vi "DecodeMonitorHeader(FHW0).vi"(11 "fhw0":u32 format="%.0x") -> (3 "FHW0":T1 {"MacID" format="%03b"})   [LabVIEW 2020, in "AIM664LV.lvlib"]
uses:
  AIM664LV.lvlib
  _controls/monitor_fhw0_type.ctl
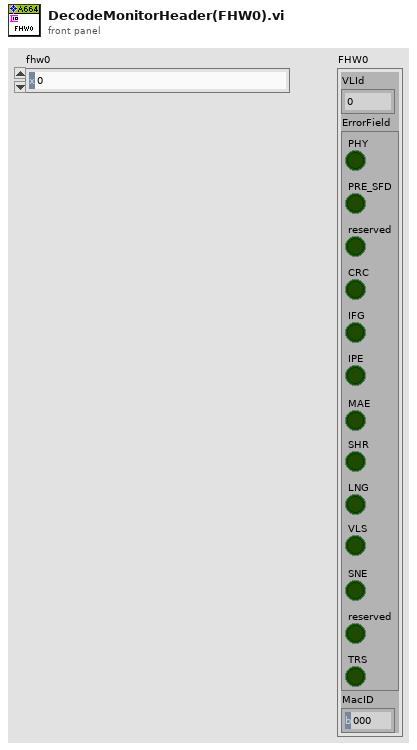
[diagram p1: front panel]
types:
  T1 = typedef "AIM664LV.lvlib/monitor_fhw0_type.ctl" = cluster{"VLId":u16, "ErrorField":cluster{"PHY":bool, "PRE_SFD":bool, "reserved":bool, "CRC":bool, "IFG":bool, "IPE":bool, "MAE":bool, "SHR":bool, "LNG":bool, "VLS":bool, "SNE":bool, "reserved":bool, "TRS":bool}, "MacID":u8}
  T2 = cluster{"Boolean array[0]":bool, "Boolean array[1]":bool, "Boolean array[2]":bool, "Boolean array[3]":bool, "Boolean array[4]":bool, "Boolean array[5]":bool, "Boolean array[6]":bool, "Boolean array[7]":bool, "Boolean array[8]":bool, "Boolean array[9]":bool, "Boolean array[10]":bool, "Boolean array[11]":bool, "Boolean array[12]":bool}
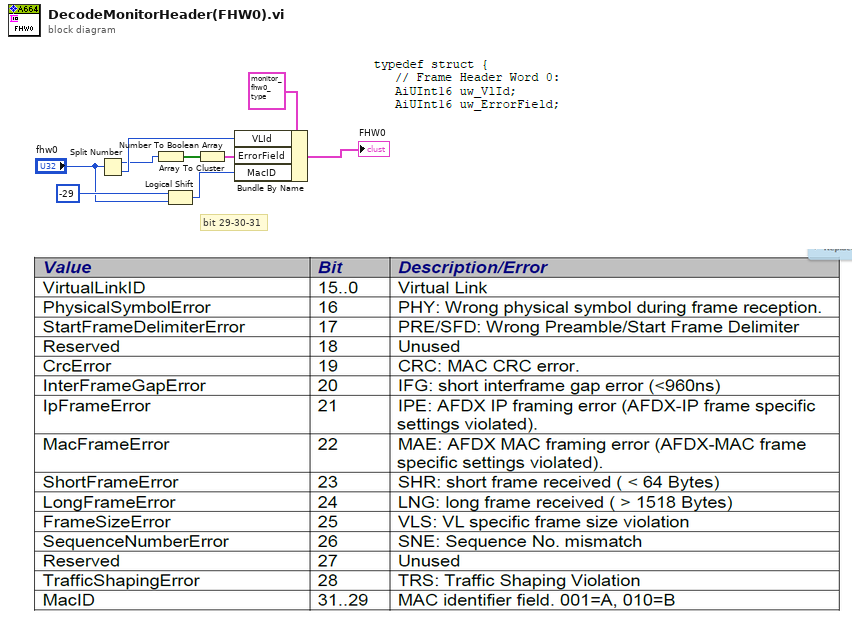
[diagram p0: block diagram]
diagram:
  # "bit 29-30-31"
  n1 = Split Number(x="fhw0") -> (hi(x)=w4:u16, lo(x)=w6:u16)
  n2 = Number To Boolean Array(number=w4) -> (Boolean array=w7:bool[])
  n3 = Logical Shift(y=i16 -29, x="fhw0") -> (x << y=w3:u32)
  n4 = Array To Cluster(array=w7) -> (cluster=w5:T2)
  n5 = Bundle By Name(cluster=T1 {"VLId"=0, "ErrorField"={"PHY"=FALSE, "PRE_SFD"=FALSE, "reserved"=FALSE, "CRC"=FALSE, "IFG"=FALSE, "IPE"=FALSE, "MAE"=FALSE, "SHR"=FALSE, "LNG"=FALSE, "VLS"=FALSE, "SNE"=FALSE, "reserved"=FALSE, "TRS"=FALSE}, "MacID"=0} ("FHW0"), "VLId"=w6, "ErrorField"=w5, "MacID"=w3) -> (→"FHW0":T1)
